vi "CSM Log Table Window.vi"(7 "Name(\"\" to use uuid)":string="Event CSM Tiny") -> ()   [LabVIEW 2020]
doc: "Template for building CSM Module without User Interface.\n\n<b>Inputs:</b>\n- <b>Name(\"\" to use uuid)</b>: Module Name\n - If Input is \"\", an uuid will be used for module name. The module is marked as stand-alone mode and will not be included in module list.\n - Fi Input end with '#', the module will worked in worker mode. Modules with the same name will shared the same message queue. Any external message will be processed by one of the modules, depends on who is free.\n - Otherwise, the input string will be used as module name, which should be unique in system. CSM will go to \"Critical Error\" state if duplicated module name is used in system.\n\n<b>Outputs:</b>\n - N/A"
uses:
  <userlib>/_NEVSTOP/Communicable State Machine(CSM)/_Support/Priority Queue/Priority Queue.lvclass/Priority Queue.ctl
  e16b33e6-092d-4751-b494-f0bfca74a912.vi
  79ee6fc1-2745-4050-a9ed-2c8a53585409.vi
  <userlib>/_NEVSTOP/Communicable State Machine(CSM)/AdvanceAPI/CSM - Revert Arguments-Safe String.vi
  <userlib>/_NEVSTOP/Communicable State Machine(CSM)/_Support/Common/Trim Single line Text.vi
  <userlib>/_NEVSTOP/Communicable State Machine(CSM)/AdvanceAPI/CSM - Break Down Multiple States String.vi
  <userlib>/_NEVSTOP/Communicable State Machine(CSM)/AdvanceAPI/CSM - Compact Multiple States.vi
  <userlib>/_NEVSTOP/Communicable State Machine(CSM)/AdvanceAPI/CSM - Make String Arguments Safe.vi
  <userlib>/_NEVSTOP/Communicable State Machine(CSM)/addons/API-String-Arugments-Support/_Support/Query Data as API String Arguments(variant).vi
  <userlib>/_NEVSTOP/Communicable State Machine(CSM)/_Support/Process/CSMP-Async Call.vi
  <userlib>/_NEVSTOP/Communicable State Machine(CSM)/_Support/GlobalEvent/GEvt-Generate Status Log.vi
  <userlib>/_NEVSTOP/Communicable State Machine(CSM)/_Support/Process/CSMP-Broadcast.vi
  <userlib>/_NEVSTOP/Communicable State Machine(CSM)/_Support/GlobalEvent/GEvt-Generate Interrupt Log.vi
  <userlib>/_NEVSTOP/Communicable State Machine(CSM)/_Support/GlobalEvent/GEvt-Generate Register Log.vi
  <userlib>/_NEVSTOP/Communicable State Machine(CSM)/_Support/Process/CSMP-Register Status.vi
  <userlib>/_NEVSTOP/Communicable State Machine(CSM)/_Support/GlobalEvent/GEvt-Generate Unregister Log.vi
  <userlib>/_NEVSTOP/Communicable State Machine(CSM)/_Support/Process/CSMP-Unregister Status.vi
  <userlib>/_NEVSTOP/Communicable State Machine(CSM)/_Support/Process/CSMP-Sync Call.vi
  <userlib>/_NEVSTOP/Communicable State Machine(CSM)/_Support/CSMQ/_CSMObj-Unlock.vi
  <userlib>/_NEVSTOP/Communicable State Machine(CSM)/_Support/Process/CSMP-PostPostMsg.vi
  <userlib>/_NEVSTOP/Communicable State Machine(CSM)/_Support/Process/CSMP-PostSendMsg.vi
  <userlib>/_NEVSTOP/Communicable State Machine(CSM)/_Support/CSMQ/_CSMObj-Lock State.vi
  <userlib>/_NEVSTOP/Communicable State Machine(CSM)/_Support/Common/Splite Reason String Part.vi
  <userlib>/_NEVSTOP/Communicable State Machine(CSM)/_Support/CSMQ/_CSMOFGV Release.vi
  <userlib>/_NEVSTOP/Communicable State Machine(CSM)/_Support/Common/Remove Comments from Line.vi
  <userlib>/_NEVSTOP/Communicable State Machine(CSM)/_Support/Common/Splite Single-line Message.vi
  <userlib>/_NEVSTOP/Communicable State Machine(CSM)/_Support/Common/Parse Next Single-line State.vi
  <userlib>/_NEVSTOP/Communicable State Machine(CSM)/_Support/CSMQ/_CSMOFGV Dequeue.vi
  <userlib>/_NEVSTOP/Communicable State Machine(CSM)/_Support/CSMQ/_CSMObj-Log Error if in a Remote Session.vi
  <userlib>/_NEVSTOP/Communicable State Machine(CSM)/_Support/GlobalEvent/GEvt-Generate State Change Log.vi
  <userlib>/_NEVSTOP/Communicable State Machine(CSM)/_Support/GlobalEvent/GEvt-Generate Remaining States Log.vi
  <userlib>/_NEVSTOP/Communicable State Machine(CSM)/_Support/GlobalEvent/GEvt-Generate Module Destroyed Log.vi
  <userlib>/_NEVSTOP/Communicable State Machine(CSM)/_Support/GlobalEvent/GEvt-Generate Complete Log.vi
  <userlib>/_NEVSTOP/Communicable State Machine(CSM)/_Support/GlobalEvent/GEvt-Generate Module Created Log.vi
  <userlib>/_NEVSTOP/Communicable State Machine(CSM)/AdvanceAPI/CSM - Keywords.vi
  <userlib>/_NEVSTOP/Communicable State Machine(CSM)/_Support/CSMQ/_CSMObj-Message Check.vi
  <userlib>/_NEVSTOP/Communicable State Machine(CSM)/_Support/CSMQ/_CSMObj-Enqueue Cross-Module Message.vi
  <userlib>/_NEVSTOP/Communicable State Machine(CSM)/_Support/CSMQ/_CSMOFGV Get.vi
  <userlib>/_NEVSTOP/Communicable State Machine(CSM)/_Support/FGV-BroadcastRegistry/Cache-Broadcast Registry Search Result.vi
  <userlib>/_NEVSTOP/Communicable State Machine(CSM)/AdvanceAPI/CSM - Register Status Change.vi
  <userlib>/_NEVSTOP/Communicable State Machine(CSM)/AdvanceAPI/CSM - Unregister Status Change.vi
  <userlib>/_NEVSTOP/Communicable State Machine(CSM)/_Support/Common/Hex Str to U8 Data.vi
  <userlib>/_NEVSTOP/Communicable State Machine(CSM)/Utility/Build Internal State String.vi
  <userlib>/_NEVSTOP/Communicable State Machine(CSM)/_Support/Common/Concatenate State with Arguments.vi
  <userlib>/_NEVSTOP/Communicable State Machine(CSM)/_Support/Common/U8 Data to Hex Str.vi
  <userlib>/_NEVSTOP/Communicable State Machine(CSM)/_Support/Priority Queue/Dequeue Element.vi
  <userlib>/_NEVSTOP/Communicable State Machine(CSM)/_Support/Priority Queue/Enqueue Element.vi
  <userlib>/_NEVSTOP/Communicable State Machine(CSM)/Utility/Trim Both Whitespace.vi
  <userlib>/_NEVSTOP/Communicable State Machine(CSM)/_Support/GlobalEvent/FGV-GlobalEventRef.vi
  <userlib>/_NEVSTOP/Communicable State Machine(CSM)/_Support/CSMQ/_CSMOFGV Obtain.vi
  <userlib>/_NEVSTOP/Communicable State Machine(CSM)/_Support/CSMQ/_CSMOFGV.vi
  <userlib>/_NEVSTOP/Communicable State Machine(CSM)/_Support/Error/CSM Not Allowed Message.vi
  <userlib>/_NEVSTOP/Communicable State Machine(CSM)/_Support/GlobalEvent/FGV-StatusChangeEventRef.vi
  <userlib>/_NEVSTOP/Communicable State Machine(CSM)/_Support/FGV-BroadcastRegistry/global-CSMQ FGV Change Flag.vi
  <userlib>/_NEVSTOP/Communicable State Machine(CSM)/_Support/FGV-BroadcastRegistry/global-Broadcast Cache Change Flag.vi
  <userlib>/_NEVSTOP/Communicable State Machine(CSM)/_Support/BroadcastRegistry/HelperVI/Broadcast Item Key.vi
  <userlib>/_NEVSTOP/Communicable State Machine(CSM)/_Support/FGV-BroadcastRegistry/FGV-BroadcastRegistry.vi
  <userlib>/_NEVSTOP/Communicable State Machine(CSM)/_Support/Message/Parse Register Message.vi
  <userlib>/_NEVSTOP/Communicable State Machine(CSM)/_Support/Message/Parse Unregister Message.vi
  <userlib>/_NEVSTOP/Communicable State Machine(CSM)/addons/API-String-Arugments-Support/_Support/Data To SingleElementsArray_with_itself_csm.vi
  <userlib>/_NEVSTOP/Communicable State Machine(CSM)/addons/API-String-Arugments-Support/_Support/Data To API String Arguments.vi
  <userlib>/_NEVSTOP/Communicable State Machine(CSM)/addons/API-String-Arugments-Support/_Support/Convert API String Arguments to Data(variant).vi
  <userlib>/_NEVSTOP/Communicable State Machine(CSM)/Communicable State Machine.lvlib
  89a8fe3c-a1f2-4f6f-a823-ce719499888a.vi
  Typedef/Def - Parsed CSMLog Line - Cluster.ctl
panel:
  in  "Table":string[][](table)
  in  "Scrollbar":i32(c297)
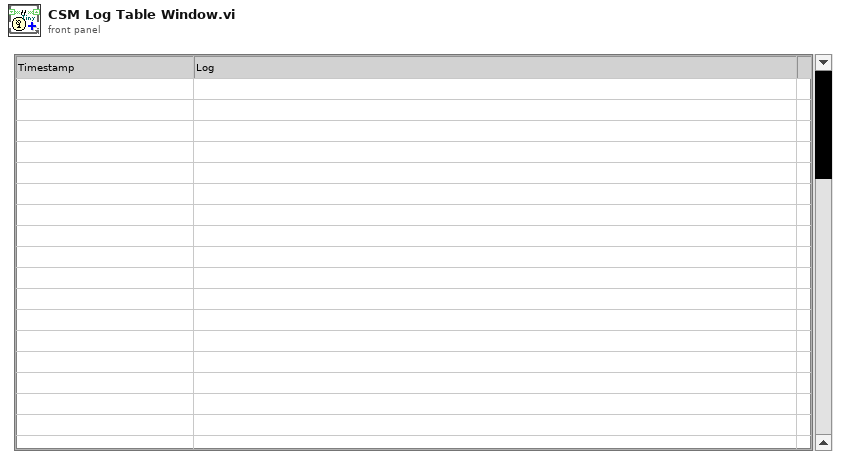
[diagram p1: front panel]
types:
  T1 = enum32{"Invalid", "Standard", "Closed", "Hidden", "Minimized", "Maximized"}
  T2 = enum32{"invalid app kind", "Development System", "Run Time System", "Student Edition", "Embedded LabVIEW", "Evaluation", "Custom"}
  T3 = typedef "Def - Parsed CSMLog Line - Cluster.ctl" = cluster{"Timestamp":timestamp, "Log Type":string, "CSM":string, "Log":string, "RawString":string}
  T4 = typedef "Communicable State Machine.lvlib/_CSM_Response Source Message.ctl" = cluster{"‘State":string, "’Arguments":string, "’Error":errorcluster}
  T5 = cluster{"Core":cluster{"Current VI Reference":refnum<vi>, "Close Panel on Exit?":bool}, "Your Boolean data":bool, "Your string data":string}
  T6 = cluster{"Current VI Reference":refnum<vi>, "Close Panel on Exit?":bool}
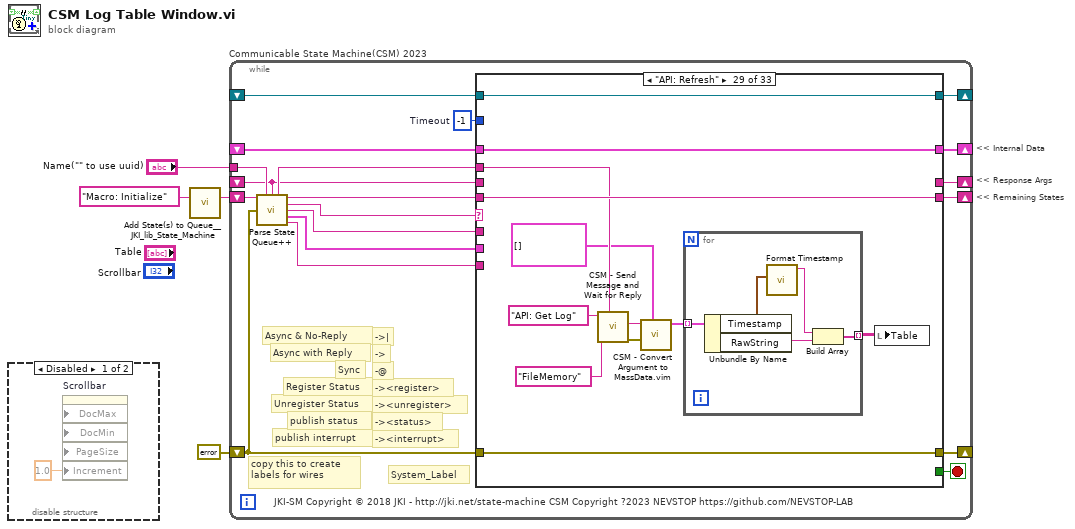
[diagram p0: block diagram]
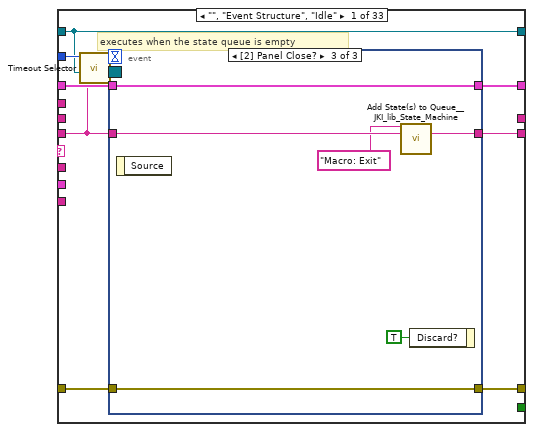
[diagram p3: hidden frame]
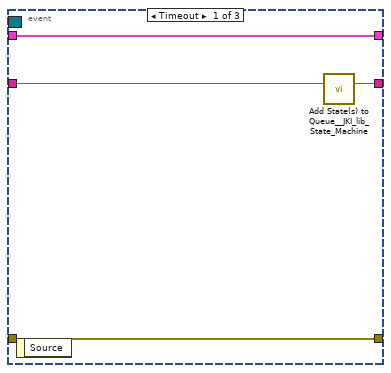
[diagram p4: hidden frame]
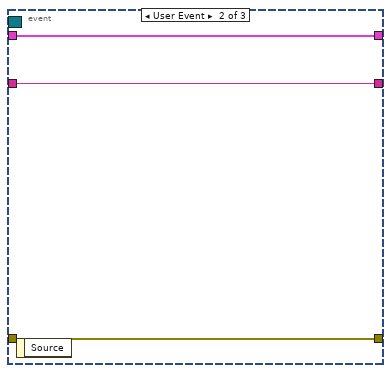
[diagram p5: hidden frame]
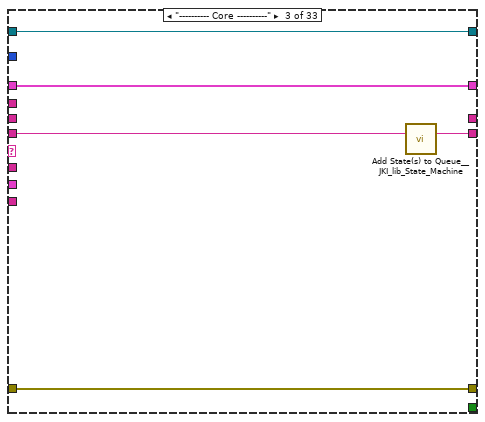
[diagram p7: hidden frame]
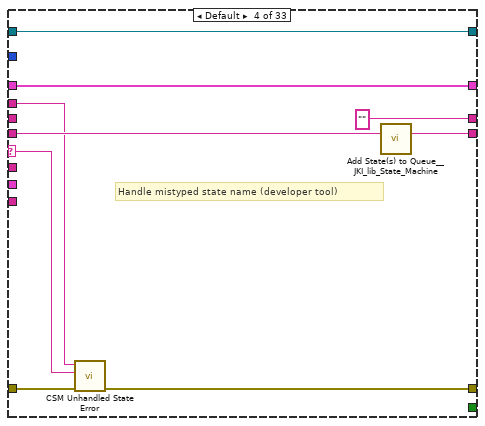
[diagram p8: hidden frame]
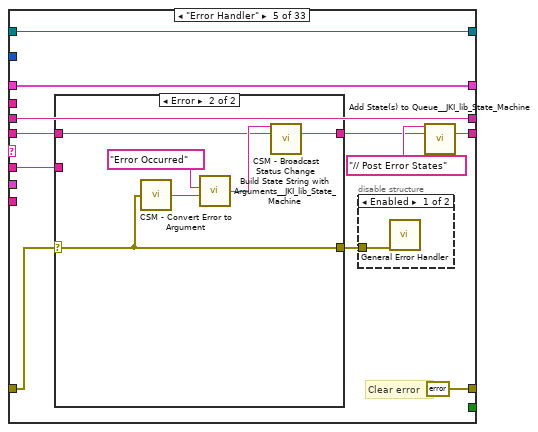
[diagram p9: hidden frame]
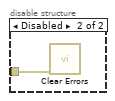
[diagram p10: hidden frame]
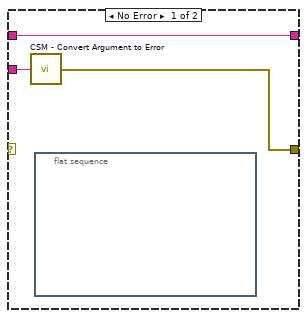
[diagram p11: hidden frame]
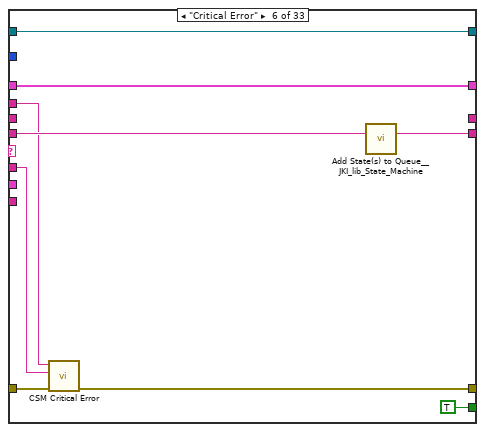
[diagram p12: hidden frame]
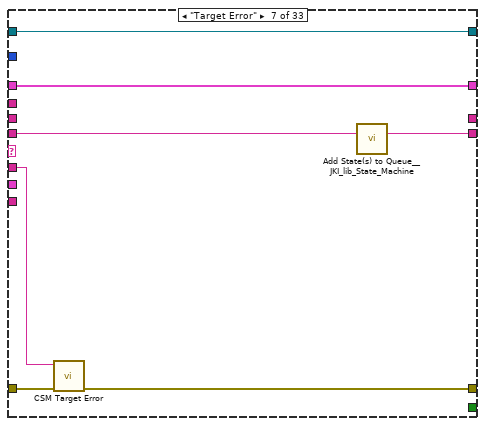
[diagram p13: hidden frame]
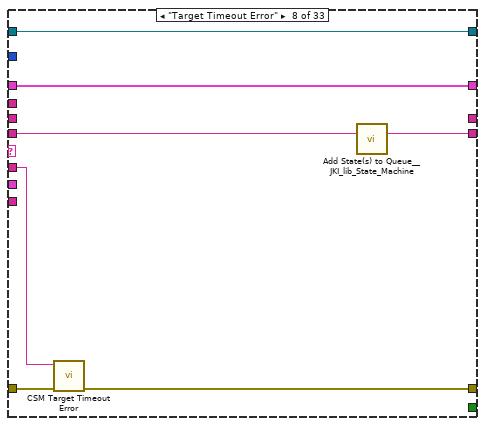
[diagram p14: hidden frame]
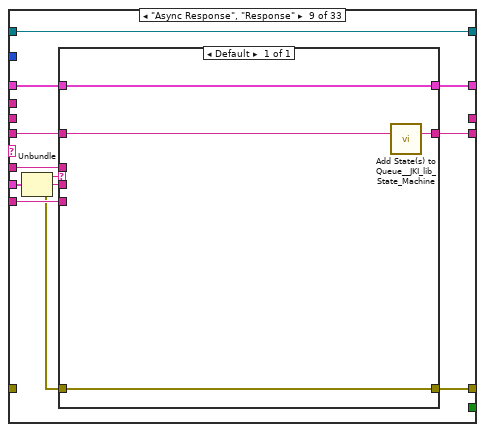
[diagram p15: hidden frame]
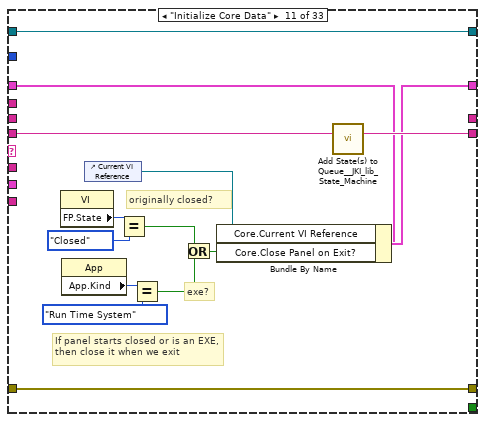
[diagram p17: hidden frame]
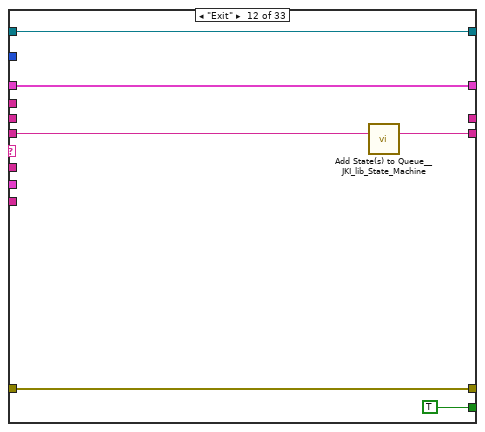
[diagram p18: hidden frame]
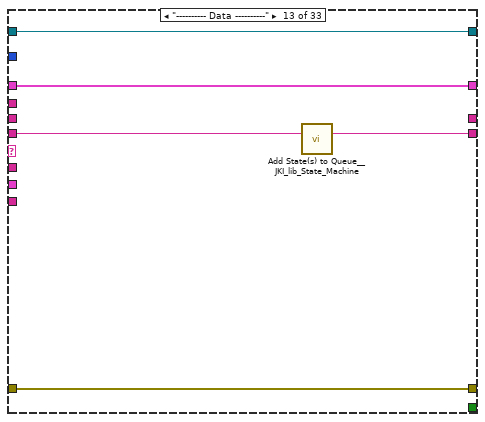
[diagram p19: hidden frame]
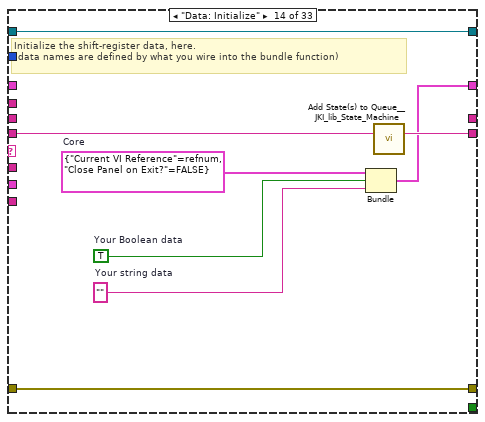
[diagram p20: hidden frame]
diagram:
  # "<< Internal Data"
  # "<< Response Args"
  # "<< Remaining States"
  n1 = disable-structure shown="Disabled" {
    frame Disabled {
      n2 = property on="Scrollbar" class="Scroll (strict)" props=["DocMax", "DocMin", "PageSize", "Increment"]("Increment"=1.0) -> ()  [unwired: 5 in, 2 out]
    }
    frame Enabled {
    }
  }
  n3 = call <vilib>:"Add State(s) to Queue__JKI_lib_State_Machine.vi"("State(s) in (\"\")"="Macro: Initialize" ("Init State(\"Macro: Initialize\")")) -> ("States Out"=w4:string)  [unwired: 14 in]
  n4 = while "Communicable State Machine(CSM) 2023" {
    shift-right: [w19] -> _
    shift-left: _ -> [w18]
    shift-right: [w22] -> _
    shift-left: errorcluster {"status"=FALSE, "code"=0, "source"=""} ("error out") -> [w16]
    shift-right: [w21] -> _
    shift-left: w4 -> [w23]
    tunnel: "Name(\"\" to use uuid)" -> [w12]
    shift-right: [w15] -> _
    shift-left: _ -> [w6]
    shift-right: [w14] -> _
    shift-left: _ -> [w13]
    stop <- w20 stop-if-true
    w17 = -1  # Timeout
    # "-><interrupt>"
    # "-><status>"
    # "-><unregister>"
    # "-><register>"
    # "-@"
    # "->"
    # "->|"
    # "publish interrupt"
    # "publish status"
    # "Unregister Status"
    # "Register Status"
    # "Sync"
    # "Async with Reply"
    # "Async & No-Reply"
    # "copy this to create labels for wires"
    # "System_Label"
    # "JKI-SM Copyright © 2018 JKI - http://jki.net/state-machine CSM Copyright ?2023 NEVSTOP https://github.com/NEVSTOP-LAB"
    n5 = call <userlib>:"Parse State Queue++.vi"("State Queue"=w23, "Name(\"\" to use uuid)"=w12, "Response Arguments"=w6, "Error In (no error)"=w16) -> ("Name Used"=w7:string, "Remaining States"=w24:string, "Current State"=w11:string, "Arguments"=w10:string, ">> Response Source Message >>"=w9:T4, ">> Source CSM >>"=w8:string)  [unwired: 6 in]
    n6 = case shown="\"API: Refresh\"" w11 {
      selector: w11 -> [_ _ _ w58 _ _ _ _ _ _ _ _ _ _ _ _ _ _ _ _ _ _ _ _ _ _ _ _ _ _ _ _ _]
      tunnel: w24 -> [w25 w49 w55 w63 w70 w93 w99 w106 w115 w128 w143 w149 w154 w162 w169 w175 w182 w187 w194 w198 w204 w209 w216 w232 w302 w308 w320 w323 w335 w346 w354 w359 w364]
      tunnel: w10 -> [_ _ _ _ w69 w88 w98 w105 w114 _ _ _ _ _ w165 w173 _ _ _ _ _ _ w211 w226 _ _ _ _ _ w343 _ _ _]
      tunnel: w18 -> [w32 w48 w52 w61 w74 w94 w101 w108 w117 w127 w136 w147 w151 _ w167 w172 w177 w184 w193 w197 w201 w207 w214 w228 w299 w305 w317 w322 w334 w345 w351 w356 w361]
      tunnel: [w31 w50 w53 w56 errorcluster {"status"=FALSE, "code"=0, "source"=""} ("error out") w89 w96 w103 w120 w129 w140 w146 w152 w159 w163 w170 w178 w185 w188 w196 w202 w206 w212 w229 w300 w306 w318 w324 w336 w347 w352 w357 w362] -> w22
      tunnel: w16 -> [w30 w50 w53 w64 w71 w95 w97 w104 _ w129 w140 w146 w152 w159 _ _ w179 w185 _ w199 w202 w206 w213 w230 w300 w306 w318 w324 w336 w347 w352 w357 w362]
      tunnel: [w33 w49 w54 w62 w66 w92 w102 w109 w116 w128 w142 w148 w153 w161 w169 w175 w181 w186 w194 w198 w203 w208 w215 w231 w301 w307 w319 w323 w335 w346 w353 w358 w363] -> w21
      tunnel: [_ _ _ _ _ TRUE _ _ _ _ _ TRUE _ _ _ _ _ _ _ _ _ _ _ _ _ _ _ _ _ _ _ _ _] -> w20
      tunnel: [w29 w48 w52 w61 w74 w94 w101 w108 w118 w127 w141 w147 w151 w160 w166 w171 w177 w184 w193 w197 w201 w207 w214 w228 w299 w305 w317 w322 w334 w345 w351 w356 w361] -> w19
      tunnel: w17 -> [w28 _ _ _ _ _ _ _ _ _ _ _ _ _ _ _ _ _ _ _ _ _ _ _ _ _ _ _ _ _ _ _ _]
      tunnel: w8 -> [_ _ _ _ _ _ _ _ w112 _ _ _ _ _ _ _ _ _ _ _ _ _ _ _ _ _ _ _ _ _ _ _ _]
      tunnel: w9 -> [_ _ _ _ _ _ _ _ w119 _ _ _ _ _ _ _ _ _ _ _ _ _ _ _ _ _ _ _ _ _ _ _ _]
      tunnel: [_ _ _ "" w65 _ _ _ _ _ _ _ _ _ w164 _ _ _ _ _ _ _ _ _ _ _ _ _ _ w342 _ _ _] -> w15
      tunnel: [w27 w47 w51 w59 w73 w90 w100 w107 w121 w126 w130 w144 w150 w155 w168 w174 w176 w183 w192 w195 w200 w205 w210 w225 w298 w303 w310 w321 w333 w344 w350 w355 w360] -> w14
      tunnel: w13 -> [w27 w47 w51 w59 w73 w90 w100 w107 w121 w126 w130 w144 w150 w155 w168 w174 w176 w183 _ w195 w200 w205 w210 w225 w298 w303 w310 w321 w333 w344 w350 w355 w360]
      tunnel: w7 -> [_ _ _ w57 _ w87 _ _ _ _ _ _ _ _ _ _ _ _ w191 _ _ _ _ _ _ _ _ _ w332 _ _ _ _]
      tunnel: w6 -> [_ _ _ _ w65 _ _ _ _ _ _ _ _ _ _ _ _ _ _ _ _ _ _ _ _ _ _ _ _ _ _ _ _]
      frame "", "Event Structure", "Idle" {
        # "executes when the state queue is empty"
        n7 = call <userlib>:"Timeout Selector.vi"("Remaining States"=w25, "Timeout Expected"=w28) -> ("Timeout"=w26:i32)  [unwired: 5 in]
        n8 = event shown="[2] Panel Close?" {
          selector: w27 -> [_ _ _]
          dyn-events: _ -> [_ _ _]
          timeout: w26 -> [_ _ _]
          tunnel: w25 -> [w37 w39 w46]
          tunnel: [w36 w39 w45] -> w33
          tunnel: w32 -> [w34 w40 w43]
          tunnel: [w35 w38 w44] -> w31
          tunnel: w30 -> [w35 w38 w44]
          tunnel: [w34 w40 w43] -> w29
          event Timeout {
            n9 = event-data() -> ()  [unwired: 1 in, 1 out]
            n10 = call <vilib>:"Add State(s) to Queue__JKI_lib_State_Machine.vi"("State(s) in (\"\")"=w37) -> ("States Out"=w36:string)  [unwired: 14 in]
          }
          event User Event {
            n11 = event-data() -> ()  [unwired: 1 in, 1 out]
          }
          event Panel Close? {
            n12 = event-data() -> ()  [unwired: 1 in, 1 out]
            n13 = call <vilib>:"Add State(s) to Queue__JKI_lib_State_Machine.vi"("State(s) in Front (\"\")"="Macro: Exit", "State(s) in (\"\")"=w46) -> ("States Out"=w45:string)  [unwired: 13 in]
            n14 = event-data("Discard?"=TRUE) -> ()  [unwired: 1 in, 1 out]
          }
        }
      }
      frame "CSM Documentation" {
      }
      frame "---------- Core ----------" {
        n15 = call <vilib>:"Add State(s) to Queue__JKI_lib_State_Machine.vi"("State(s) in (\"\")"=w55) -> ("States Out"=w54:string)  [unwired: 14 in]
      }
      frame Default {
        # "Handle mistyped state name (developer tool)"
        n16 = call <userlib>:"CSM Unhandled State Error.vi"("error in (no error)"=w64, "State"=w58, "CSM"=w57) -> ("error out"=w56:errorcluster)  [unwired: 8 in]
        n17 = call <vilib>:"Add State(s) to Queue__JKI_lib_State_Machine.vi"("State(s) in (\"\")"=w63) -> ("States Out"=w62:string)  [unwired: 14 in]
      }
      frame "Error Handler" {
        # "Clear error"
        n18 = case shown="Error" w71 {
          selector: w71 -> [_ w81]
          tunnel: [w80 w83] -> w67
          tunnel: w70 -> [w80 w82]
          tunnel: w69 -> [w79 _]
          tunnel: [w78 w81] -> w72
          frame No Error {
            n19 = call <userlib>:"CSM - Convert Argument to Error.vi"("Argument"=w79) -> ("error"=w78:errorcluster)  [unwired: 4 in]
            n20 = flat-sequence {
              frame #0 {
              }
            }
          }
          frame Error {
            n21 = call <userlib>:"CSM - Convert Error to Argument.vi"("error in (no error)"=w81) -> ("Arguments"=w85:string)  [unwired: 4 in]
            n22 = call <vilib>:"Build State String with Arguments__JKI_lib_State_Machine.vi"("Arguments (\"\")"=w85, "State"="Error Occurred" ("Status with Arguments")) -> ("State with Arguments"=w84:string)  [unwired: 4 in]
            n23 = call <userlib>:"CSM - Broadcast Status Change.vi"("Status with Arguments"=w84, "State Queue"=w82) -> ("Remaining States"=w83:string)  [unwired: 13 in]
          }
        }
        n24 = disable-structure shown="Enabled" {
          disable-tunnel: w72 -> [w76 w77]
          frame Enabled {
            n25 = call <vilib>:"General Error Handler.vi"("error in (no error)"=w76) -> ()  [unwired: 10 in, 5 out]
          }
          frame Disabled {
            n26 = call <vilib>:"Clear Errors.vi"("error in (no error)"=w77) -> ()  [unwired: 5 in, 2 out]
          }
        }
        n27 = call <vilib>:"Add State(s) to Queue__JKI_lib_State_Machine.vi"("State(s) in Front (\"\")"="// Post Error States", "State(s) in (\"\")"=w67) -> ("States Out"=w66:string)  [unwired: 13 in]
      }
      frame "Critical Error" {
        n28 = call <userlib>:"CSM Critical Error.vi"("error in (no error)"=w95, "input"=w88, "CSM Name"=w87) -> ("error out"=w89:errorcluster)  [unwired: 8 in]
        n29 = call <vilib>:"Add State(s) to Queue__JKI_lib_State_Machine.vi"("State(s) in (\"\")"=w93) -> ("States Out"=w92:string)  [unwired: 14 in]
      }
      frame "Target Error" {
        n30 = call <userlib>:"CSM Target Error.vi"("error in (no error)"=w97, "CSM Name"=w98) -> ("error out"=w96:errorcluster)  [unwired: 9 in]
        n31 = call <vilib>:"Add State(s) to Queue__JKI_lib_State_Machine.vi"("State(s) in (\"\")"=w99) -> ("States Out"=w102:string)  [unwired: 14 in]
      }
      frame "Target Timeout Error" {
        n32 = call <userlib>:"CSM Target Timeout Error.vi"("error in (no error)"=w104, "CSM Name"=w105) -> ("error out"=w103:errorcluster)  [unwired: 9 in]
        n33 = call <vilib>:"Add State(s) to Queue__JKI_lib_State_Machine.vi"("State(s) in (\"\")"=w106) -> ("States Out"=w109:string)  [unwired: 14 in]
      }
      frame "Async Response", "Response" {
        n34 = Unbundle(w119) -> ("‘State"=w113:string, "’Arguments"=w111:string, "’Error"=w110:errorcluster)
        n35 = case shown="Default" w113 {
          tunnel: [w125] -> w120
          tunnel: w110 -> [w125]
          tunnel: [w124] -> w118
          tunnel: w117 -> [w124]
          tunnel: [w122] -> w116
          tunnel: w115 -> [w123]
          tunnel: w114 -> [_]
          tunnel: w112 -> [_]
          tunnel: w111 -> [_]
          frame Default {
            n36 = call <vilib>:"Add State(s) to Queue__JKI_lib_State_Machine.vi"("State(s) in (\"\")"=w123) -> ("States Out"=w122:string)  [unwired: 14 in]
          }
        }
      }
      frame "Async Message Posted" {
      }
      frame "Initialize Core Data" {
        # "originally closed?"
        # "exe?"
        # "If panel starts closed or is an EXE, then close it when we exit"
        n37 = property class="VI"() -> ("FP.State"=w133:T1)  [unwired: 2 in, 2 out]
        n38 = property class="App"() -> ("App.Kind"=w139:T2)  [unwired: 2 in, 2 out]
        n39 = control-ref of="Current VI Reference"() -> (w134:refnum<vi>)
        n40 = Equal?(x=w133, y=T1."Closed" ("Front Panel Window:State")) -> (x = y?=w131:bool)
        n41 = Equal?(x=w139, y=T2."Run Time System" ("Application:Kind")) -> (x = y?=w137:bool)
        n42 = Or(x=w131, y=w137) -> (x .or. y?=w135:bool)
        n43 = Bundle By Name(cluster=w136, "Core.Current VI Reference"=w134, "Core.Close Panel on Exit?"=w135) -> (w141:T5)
        n44 = call <vilib>:"Add State(s) to Queue__JKI_lib_State_Machine.vi"("State(s) in (\"\")"=w143) -> ("States Out"=w142:string)  [unwired: 14 in]
      }
      frame "Exit" {
        n45 = call <vilib>:"Add State(s) to Queue__JKI_lib_State_Machine.vi"("State(s) in (\"\")"=w149) -> ("States Out"=w148:string)  [unwired: 14 in]
      }
      frame "---------- Data ----------" {
        n46 = call <vilib>:"Add State(s) to Queue__JKI_lib_State_Machine.vi"("State(s) in (\"\")"=w154) -> ("States Out"=w153:string)  [unwired: 14 in]
      }
      frame "Data: Initialize" {
        w156 = T6 {"Current VI Reference"=refnum, "Close Panel on Exit?"=FALSE}  # Core
        w158 = TRUE  # Your Boolean data
        w157 = ""  # Your string data
        # "Initialize the shift-register data, here.\n(data names are defined by what you wire into the bundle function)"
        n47 = Bundle("Core"=w156, "Your Boolean data"=w158, "Your string data"=w157) -> (w160:T5)  [unwired: 1 in]
        n48 = call <vilib>:"Add State(s) to Queue__JKI_lib_State_Machine.vi"("State(s) in (\"\")"=w162) -> ("States Out"=w161:string)  [unwired: 14 in]
      }
      frame "Data: Get Configuration", "Data: Get Internal Data" {
        n49 = call "Query Data as API String Arguments.vim"("Setting Name"=w165, "Internal Data"=w167) -> ("error"=w163:errorcluster, "Setting as String"=w164:string, "Internal Data(dup)"=w166:T5)  [unwired: 7 in]
      }
      frame "Data: Set Configuration" {
        n50 = call "Convert API String Arguments to Data.vim"("Type"=w172, "String"=w173) -> ("error"=w170:errorcluster, "Data"=w171:T5)  [unwired: 6 in]
      }
      frame "Data: Cleanup" {
        # "Cleanup any data and references, here.\n(this is called automatically, by the Macro: Exit)"
        n51 = Unbundle By Name(w177) -> ("Core.Current VI Reference"=w180:refnum<vi>)
        n52 = Close Reference(reference=w180, error in (no error)=w179) -> (error out=w178:errorcluster)
        n53 = call <vilib>:"Add State(s) to Queue__JKI_lib_State_Machine.vi"("State(s) in (\"\")"=w182) -> ("States Out"=w181:string)  [unwired: 14 in]
      }
      frame "---------- Events ----------" {
        n54 = call <vilib>:"Add State(s) to Queue__JKI_lib_State_Machine.vi"("State(s) in (\"\")"=w187) -> ("States Out"=w186:string)  [unwired: 14 in]
      }
      frame "Events: Register" {
        n55 = call <userlib>:"CSM - Get New State Notifier Event.vi"("Name(\"\" to use uuid) in"=w191) -> ("Error out"=w189:errorcluster, "New State Notifier Event"=w190:refnum<user-event>)  [unwired: 9 in]
        n56 = register-events(error in=w189, w190) -> (reference out=w192:refnum<event-registration>, error out=w188:errorcluster)  [unwired: 1 in]
      }
      frame "Events: Unregister" {
        n57 = Unregister For Events(event registration refnum=w195, error in=w199) -> (error out=w196:errorcluster)
      }
      frame "---------- UI ----------" {
        n58 = call <vilib>:"Add State(s) to Queue__JKI_lib_State_Machine.vi"("State(s) in (\"\")"=w204) -> ("States Out"=w203:string)  [unwired: 14 in]
      }
      frame "UI: Initialize" {
        n59 = call <vilib>:"Add State(s) to Queue__JKI_lib_State_Machine.vi"("State(s) in (\"\")"=w209) -> ("States Out"=w208:string)  [unwired: 14 in]
      }
      frame "UI: Cursor Set" {
        # "Argument"
        n60 = disable-structure shown="TARGET_TYPE!=Windows" {
          disable-tunnel: w213 -> [w219 w224]
          disable-tunnel: [w218 w224] -> w212
          disable-tunnel: w211 -> [w217 _]
          frame condition #0 (active) {
            n61 = case shown="\"Idle\", Default" w217 {
              tunnel: w219 -> [w221 w223]
              tunnel: [w220 w222] -> w218
              frame "Idle", Default {
                n62 = call <vilib>:"Unset Busy.vi"("error in (no error)"=w221) -> ("error out"=w220:errorcluster)  [unwired: 10 in]
              }
              frame "Busy" {
                n63 = call <vilib>:"Set Busy.vi"("error in (no error)"=w223) -> ("error out"=w222:errorcluster)  [unwired: 9 in, 1 out]
              }
            }
          }
          frame condition #1 {
          }
        }
        n64 = call <vilib>:"Add State(s) to Queue__JKI_lib_State_Machine.vi"("State(s) in (\"\")"=w216) -> ("States Out"=w215:string)  [unwired: 14 in]
      }
      frame "UI: Front Panel State" {
        # "Argument"
        n65 = Unbundle By Name(w228) -> ("Core.Current VI Reference"=w227:refnum<vi>)
        n66 = call <vilib>:"Add State(s) to Queue__JKI_lib_State_Machine.vi"("State(s) in (\"\")"=w232) -> ("States Out"=w231:string)  [unwired: 14 in]
        n67 = case shown="\"Close\", \"Closed\"" w226 {
          tunnel: w230 -> [w238 w253 w264 w277 w290]
          tunnel: [w240 w254 w266 w279 w292] -> w229
          tunnel: w227 -> [w239 w251 w265 w278 w291]
          frame "Open", "Standard", Default {
            w233 = T1."Standard" ("State")
            n68 = property class="VI"(reference=w239, error in=w238) -> (reference out=w236:refnum<vi>, error out=w237:errorcluster, "FP.State"=w235:T1)
            n69 = Not Equal?(x=w235, y=w233) -> (x != y?=w234:bool)
            n70 = case shown="True" w234 {
              tunnel: [w244 w246] -> w240
              tunnel: w237 -> [w243 w246]
              tunnel: w236 -> [w242 _]
              tunnel: w233 -> [w241 _]
              frame True {
                n71 = invoke class="VI" method="FP.Open"(reference=w242, error in=w243, "Activate"=TRUE, "State"=w241) -> (error out=w244:errorcluster)  [unwired: 1 in, 4 out]
              }
              frame False {
              }
            }
          }
          frame "Close", "Closed" {
            n72 = property class="VI"(reference=w251, error in=w253) -> (reference out=w250:refnum<vi>, error out=w252:errorcluster, "FP.State"=w248:T1)
            n73 = Not Equal?(x=w248, y=T1."Closed" ("Front Panel Window:State")) -> (x != y?=w247:bool)
            n74 = case shown="False" w247 {
              tunnel: [w255 w258] -> w254
              tunnel: w252 -> [w255 w257]
              tunnel: w250 -> [_ w256]
              frame False {
              }
              frame True {
                n75 = invoke class="VI" method="FP.Close"(reference=w256, error in=w257) -> (error out=w258:errorcluster)  [unwired: 1 in, 2 out]
              }
            }
          }
          frame "Hidden", "Hide" {
            w259 = T1."Hidden" ("State")
            n76 = property class="VI"(reference=w265, error in=w264) -> (reference out=w262:refnum<vi>, error out=w263:errorcluster, "FP.State"=w261:T1)
            n77 = Not Equal?(x=w261, y=w259) -> (x != y?=w260:bool)
            n78 = case shown="True" w260 {
              tunnel: [w270 w271] -> w266
              tunnel: w263 -> [w269 w271]
              tunnel: w262 -> [w268 _]
              tunnel: w259 -> [w267 _]
              frame True {
                n79 = invoke class="VI" method="FP.Open"(reference=w268, error in=w269, "State"=w267) -> (error out=w270:errorcluster)  [unwired: 2 in, 4 out]
              }
              frame False {
              }
            }
          }
          frame "Minimize", "Minimized" {
            w272 = T1."Minimized" ("State")
            n80 = property class="VI"(reference=w278, error in=w277) -> (reference out=w275:refnum<vi>, error out=w276:errorcluster, "FP.State"=w274:T1)
            n81 = Not Equal?(x=w274, y=w272) -> (x != y?=w273:bool)
            n82 = case shown="True" w273 {
              tunnel: [w283 w284] -> w279
              tunnel: w276 -> [w282 w284]
              tunnel: w275 -> [w281 _]
              tunnel: w272 -> [w280 _]
              frame True {
                n83 = invoke class="VI" method="FP.Open"(reference=w281, error in=w282, "State"=w280) -> (error out=w283:errorcluster)  [unwired: 2 in, 4 out]
              }
              frame False {
              }
            }
          }
          frame "Maximize", "Maximized" {
            w285 = T1."Maximized" ("State")
            n84 = property class="VI"(reference=w291, error in=w290) -> (reference out=w288:refnum<vi>, error out=w289:errorcluster, "FP.State"=w287:T1)
            n85 = Not Equal?(x=w287, y=w285) -> (x != y?=w286:bool)
            n86 = case shown="True" w286 {
              tunnel: [w296 w297] -> w292
              tunnel: w289 -> [w295 w297]
              tunnel: w288 -> [w294 _]
              tunnel: w285 -> [w293 _]
              frame True {
                n87 = invoke class="VI" method="FP.Open"(reference=w294, error in=w295, "State"=w293) -> (error out=w296:errorcluster)  [unwired: 2 in, 4 out]
              }
              frame False {
              }
            }
          }
        }
      }
      frame "---------- Macro ----------" {
        n88 = call <vilib>:"Add State(s) to Queue__JKI_lib_State_Machine.vi"("State(s) in (\"\")"=w302) -> ("States Out"=w301:string)  [unwired: 14 in]
      }
      frame "Macro: Initialize" {
        w304 = "Data: Initialize\nInitialize Core Data\nEvents: Register\nUI: Initialize\n//UI: Front Panel State >> Open"  # Data: Initialize Initialize Core Data Events: Register UI: Initialize //UI: Front Panel State >> Open
        n89 = call <vilib>:"Add State(s) to Queue__JKI_lib_State_Machine.vi"("State(s) in Front (\"\")"=w304, "State(s) in (\"\")"=w308) -> ("States Out"=w307:string)  [unwired: 13 in]
      }
      frame "Macro: Exit" {
        n90 = Unbundle By Name(w317) -> ("Core.Close Panel on Exit?"=w316:bool)
        n91 = Select(t="UI: Front Panel State >> Close", s=w316, f="") -> (s? t:f=w313:string)
        n92 = call <vilib>:"Add State(s) to Queue__JKI_lib_State_Machine.vi"("State(s) in Front (\"\")"="//Exit Sub-Modules ", "State(s) in (\"\")"=w313, "State(s) at Back (\"\")"="Data: Cleanup\nEvents: Unregister\nExit") -> ("States Out"=w311:string)  [unwired: 12 in]
        n93 = call <vilib>:"Add State(s) to Queue__JKI_lib_State_Machine.vi"("State(s) in Front (\"\")"=w311, "State(s) in (\"\")"=w320) -> ("States Out"=w319:string)  [unwired: 13 in]
      }
      frame "---------- API ----------" {
      }
      frame "API: Refresh" {
        n94 = call <userlib>:"CSM - Send Message and Wait for Reply.vi"("Current Module(\"\" to generate a ID)"=w332, "Target Module"="FileMemory", "State"="API: Get Log") -> ("error out"=w328:errorcluster, "Arguments"=w329:string)  [unwired: 6 in, 1 out]
        n95 = call "CSM - Convert Argument to MassData.vim"("Type"=T3[] [] ("subarray"), "error in (no error)"=w328, "MassData Argument"=w329) -> ("Data"=w326:T3[])  [unwired: 5 in, 1 out]
        n96 = for {
          tunnel: w326 -> [w341] mode=indexing
          tunnel: [w337] -> w325 mode=indexing
          n97 = Unbundle By Name(w341) -> ("Timestamp"=w339:timestamp, "RawString"=w340:string)
          n98 = call <userlib>:"Format Timestamp.vi"("timestamp"=w339) -> ("String"=w338:string)  [unwired: 10 in]
          n99 = Build Array(w338, w340) -> (w337:string[])
        }
        n100 = local write "Table"(w325) -> ()
      }
      frame "API: API2" {
        # "unpack Hex String  to Variant\nif complex parameter is needed."
        n101 = call <userlib>:"CSM - Convert HexStr to Data.vi"("HEX String"=w343) -> ()  [unwired: 7 in, 2 out]
        n102 = disable-structure shown="Disabled" {
          disable-tunnel: [w348 "API2 Response"] -> w342
          frame Disabled {
            # "pack variant to hexstr \nif complex response is needed."
            # "complex Response"
            n103 = call <userlib>:"CSM - Convert Data to HexStr.vi"() -> ("HEX String (0-9,A-F)"=w348:string)  [unwired: 9 in]
          }
          frame Enabled {
          }
        }
      }
      frame "---------- Action ----------" {
        n104 = call <vilib>:"Add State(s) to Queue__JKI_lib_State_Machine.vi"("State(s) in (\"\")"=w354) -> ("States Out"=w353:string)  [unwired: 14 in]
      }
      frame "Action: action1" {
        n105 = call <vilib>:"Add State(s) to Queue__JKI_lib_State_Machine.vi"("State(s) in (\"\")"=w359) -> ("States Out"=w358:string)  [unwired: 14 in]
      }
      frame "Action: action2" {
        n106 = call <vilib>:"Add State(s) to Queue__JKI_lib_State_Machine.vi"("State(s) in (\"\")"=w364) -> ("States Out"=w363:string)  [unwired: 14 in]
      }
    }
  }
